vi "sort sequence template 1.vi"(8 "error in":errorcluster) -> (3 "cycle results cluster out":T1, 11 "cycle results cluster IN":T1)   [LabVIEW 2016]
doc: "Takes a sample type and sorts by sequence"
uses:
  controls/cycle results control.ctl
  <vilib>/Analysis/baseanly.llb/Mean (DBL).vi
  <vilib>/Analysis/NI_AALBase.lvlib
panel:
  out "error out":errorcluster
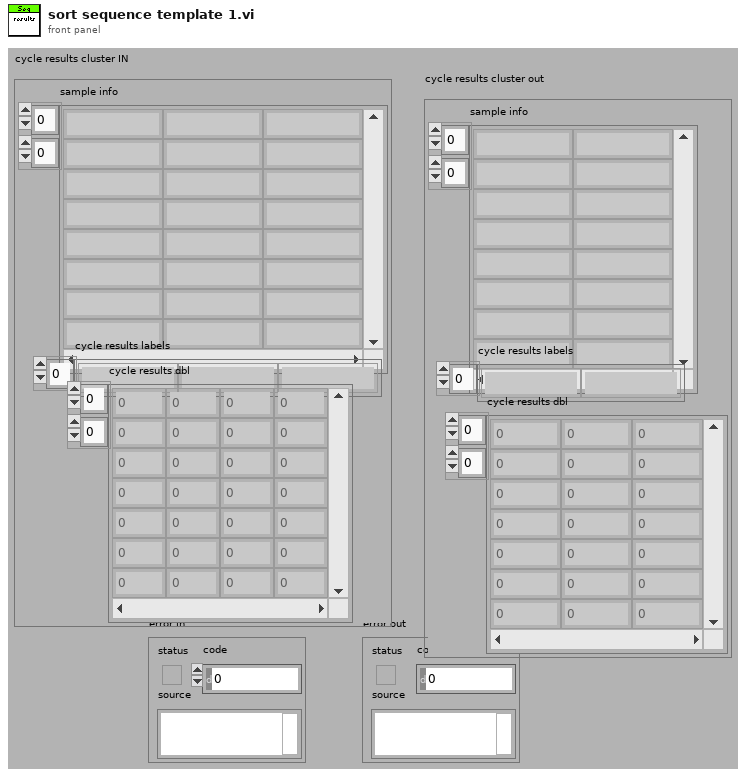
[diagram p1: front panel]
types:
  T1 = typedef "cycle results control.ctl" = cluster{"sample info":string[][], "cycle results labels":string[], "cycle results dbl":dbl[][]}
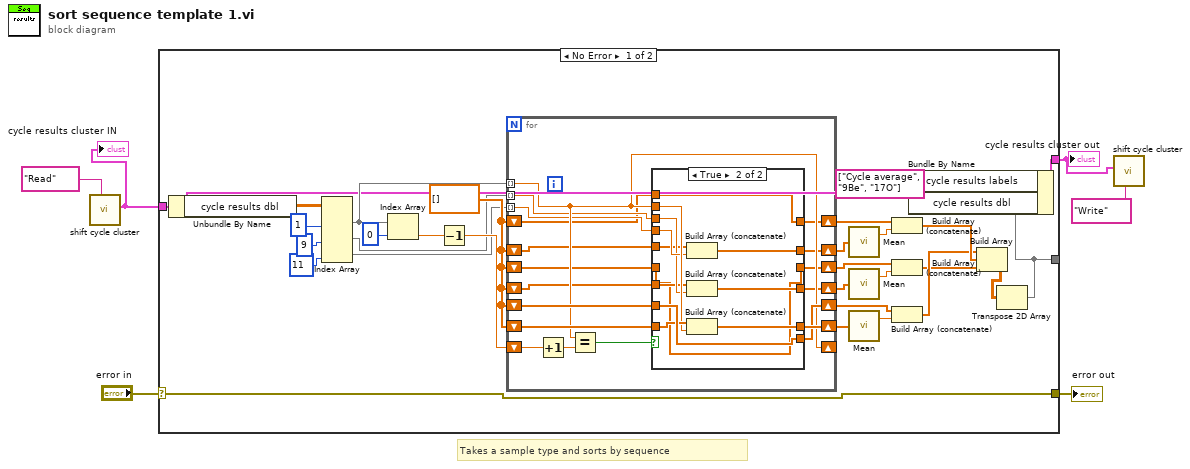
[diagram p0: block diagram]
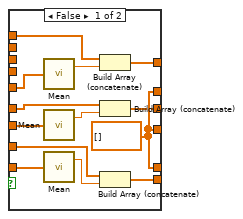
[diagram p2: hidden frame]
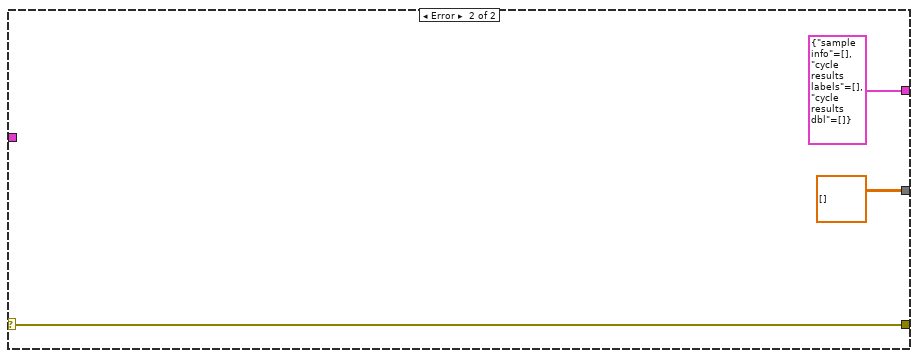
[diagram p3: hidden frame]
diagram:
  # "Takes a sample type and sorts by sequence"
  n1 = call "shift cycle cluster.vi"("read write shift"="Read") -> ("cycle results cluster out"=w1:T1)  [unwired: 9 in, 1 out]
  "cycle results cluster IN" <- w1
  n2 = case shown="No Error" "error in" {
    selector: "error in" -> [w12 w80]
    tunnel: w1 -> [w11 _]
    tunnel: [w7 dbl[][] []] -> _
    tunnel: [w9 T1 {"sample info"=[], "cycle results labels"=[], "cycle results dbl"=[]} ("cycle results cluster IN")] -> w3
    tunnel: [w12 w80] -> w5
    frame No Error {
      w25 = dbl[] []
      n3 = Unbundle By Name(w11) -> ("cycle results dbl"=w22:dbl[][])
      n4 = Index Array(array=w22, index (col) #1=1 ("disabled index (col)"), index (col) #2=9 ("index (col)"), index (col) #3=11 ("index (col)")) -> (element #1=w18:dbl[], element #2=w17:dbl[], element #3=w16:dbl[])  [unwired: 3 in]
      n5 = Index Array(array=w18, index=0) -> (element=w26:dbl)
      n6 = Decrement(x=w26) -> (x-1=w24:dbl)
      n7 = for {
        tunnel: w18 -> [w47] mode=indexing
        shift-right: [w51] -> w28
        shift-left: w25 -> [w50]
        shift-right: [w49] -> w35
        shift-left: w25 -> [w48]
        shift-right: [w47] -> _
        shift-left: w24 -> [w53]
        tunnel: w16 -> [w46] mode=indexing
        tunnel: w17 -> [w45] mode=indexing
        shift-right: [w44] -> w27
        shift-left: w25 -> [w41]
        shift-right: [w43] -> w29
        shift-left: w25 -> [w42]
        shift-right: [w40] -> w30
        shift-left: w25 -> [w38]
        shift-right: [w39] -> w33
        shift-left: w25 -> [w37]
        n8 = Increment(x=w53) -> (x+1=w36:dbl)
        n9 = Equal?(x=w47, y=w36) -> (x = y?=w52:bool)
        n10 = case shown="True" w52 {
          tunnel: w47 -> [_ w75]
          tunnel: [w58 w78] -> w51
          tunnel: w50 -> [w66 w76]
          tunnel: [w65 w77] -> w49
          tunnel: w48 -> [w64 w77]
          tunnel: w46 -> [_ w74]
          tunnel: w45 -> [_ w73]
          tunnel: [w58 w72] -> w44
          tunnel: [w58 w71] -> w43
          tunnel: w42 -> [w60 w70]
          tunnel: w41 -> [w59 w69]
          tunnel: [w57 w68] -> w40
          tunnel: [w56 w67] -> w39
          tunnel: w38 -> [w55 w68]
          tunnel: w37 -> [w54 w67]
          frame False {
            w58 = dbl[] []
            n11 = call-poly <vilib>:"Mean.vi"("X"=w60) -> ("mean"=w61:dbl)  [unwired: 1 out]
            n12 = call-poly <vilib>:"Mean.vi"("X"=w59) -> ("mean"=w62:dbl)  [unwired: 1 out]
            n13 = call-poly <vilib>:"Mean.vi"("X"=w66) -> ("mean"=w63:dbl)  [unwired: 1 out]
            n14 = Build Array (concatenate)(w55, w61) -> (w57:dbl[])
            n15 = Build Array (concatenate)(w54, w62) -> (w56:dbl[])
            n16 = Build Array (concatenate)(w64, w63) -> (w65:dbl[])
          }
          frame True {
            n17 = Build Array (concatenate)(w70, w74) -> (w71:dbl[])
            n18 = Build Array (concatenate)(w69, w73) -> (w72:dbl[])
            n19 = Build Array (concatenate)(w76, w75) -> (w78:dbl[])
          }
        }
      }
      n20 = call-poly <vilib>:"Mean.vi"("X"=w29) -> ("mean"=w31:dbl)  [unwired: 1 out]
      n21 = call-poly <vilib>:"Mean.vi"("X"=w27) -> ("mean"=w32:dbl)  [unwired: 1 out]
      n22 = call-poly <vilib>:"Mean.vi"("X"=w28) -> ("mean"=w34:dbl)  [unwired: 1 out]
      n23 = Build Array (concatenate)(w30, w31) -> (w15:dbl[])
      n24 = Build Array (concatenate)(w33, w32) -> (w13:dbl[])
      n25 = Build Array (concatenate)(w35, w34) -> (w14:dbl[])
      n26 = Build Array(w14, w15, w13) -> (w8:dbl[][])
      n27 = Transpose 2D Array(2D array=w8) -> (transposed array=w7:dbl[][])
      n28 = Bundle By Name(cluster=w11, "cycle results labels"=string[] ["Cycle average", "9Be", "17O"], "cycle results dbl"=w7) -> (w9:T1)
    }
    frame Error {
    }
  }
  "error out" <- w5
  "cycle results cluster out" <- w3
  n29 = call "shift cycle cluster.vi"("read write shift"="Write", "cycle results cluster In"=w3) -> ()  [unwired: 8 in, 2 out]
